vi "Timing_Main.vi"(8 "error in (no error)":errorcluster) -> (0 "error out":errorcluster)   [LabVIEW 2013]
doc: "This is Top Level VI for Timing Module. You can communicate with this module using its API. Communication is made based on queue. This module has not User Interface so I chase State Machine architecture."
uses:
  General/Controls/#TD_General_CommunicationQueueStates_Enum.ctl
  Private controls/#TD_Timing_InnerData_Cluster.ctl
  Private controls/#TD_Timing_ModuleStates_Enum.ctl
  Private controls/#TD_Timing_ModuleData_Cluster.ctl
  General/Controls/#TD_General_FromWho_Enum.ctl
  Private controls/#TD_Timing_Timers_Enum.ctl
  Private controls/#TD_Timing_TimerData_Cluster.ctl
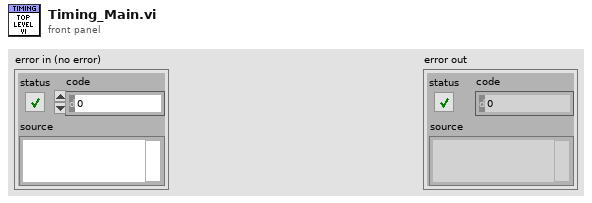
[diagram p1: front panel]
types:
  T1 = typedef "#TD_General_CommunicationQueueStates_Enum.ctl" = enum16{"ERROR_Default", "Obtain", "GetRef", "Enqueue", "EnqueueAtOpp", "GetStatus", "Release"}
  T2 = typedef "#TD_General_FromWho_Enum.ctl" = enum16{"ERROR_Default", "UserConsole", "DisplayConsole", "SensorInterface", "Controller", "Database", "Timing", "ErrorHandling"}
  T3 = typedef "#TD_Timing_ModuleStates_Enum.ctl" = enum16{"ERROR_Default", "Init", "Close", "ErrorHandling", "ResetTimer", "CheckTime", "StopTiming"}
  T4 = typedef "#TD_Timing_ModuleData_Cluster.ctl" = cluster{"Action":T3, "Data":variant}
  T5 = typedef "#TD_General_IntermoduleData_Cluster.ctl" = cluster{"Sender":T2, "ModuleData":variant}
  T6 = typedef "#TD_Timing_InnerData_Cluster.ctl" = cluster{"Sth":bool, "TimersData":T7[]}
  T7 = typedef "#TD_Timing_TimerData_Cluster.ctl" = cluster{"Timer":T8, "StartTime":timestamp, "TimeToMach":dbl, "Count?":bool}
  T8 = typedef "#TD_Timing_Timers_Enum.ctl" = enum16{"Timer_01"}
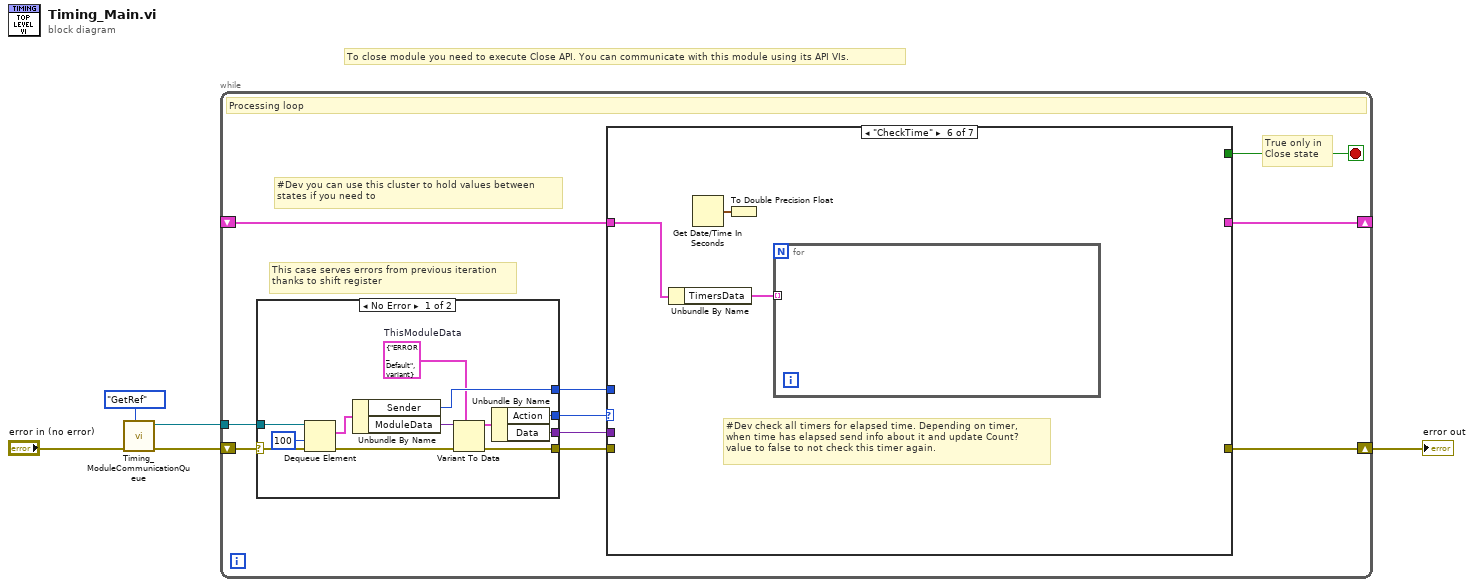
[diagram p0: block diagram]
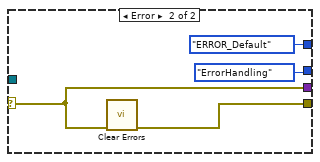
[diagram p2: hidden frame]
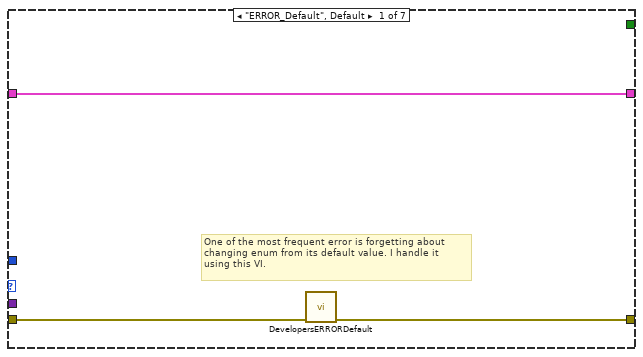
[diagram p3: hidden frame]
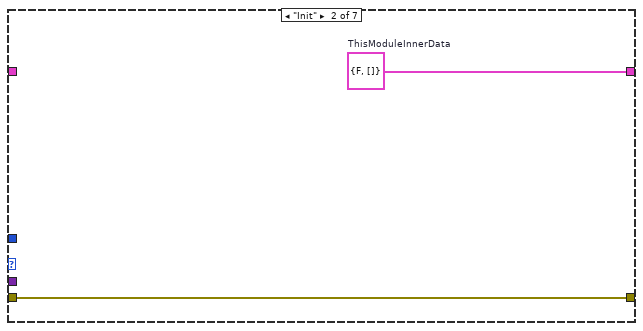
[diagram p4: hidden frame]
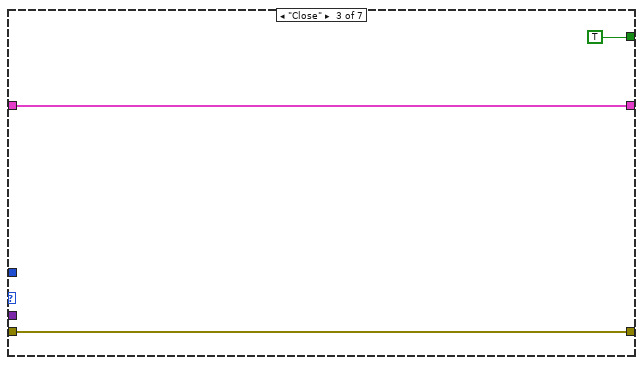
[diagram p5: hidden frame]
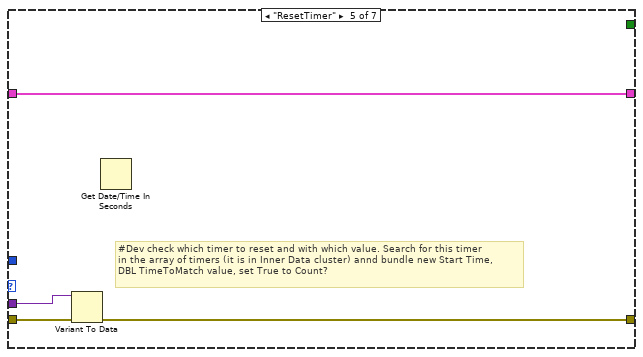
[diagram p7: hidden frame]
diagram:
  # "To close module you need to execute Close API. You can communicate with this module using its API VIs."
  n1 = call "Timing_ModuleCommunicationQueue.vi"("Action"=#TD_General_CommunicationQueueStates_Enum."GetRef", "error in (no error)"="error in (no error)") -> ("error out"=w2:errorcluster, "Ref out"=w3:refnum<queue>)  [unwired: 7 in, 1 out]
  n2 = while {
    tunnel: w3 -> [w14]
    shift-right: [w7] -> w1
    shift-left: w2 -> [w15]
    shift-right: [w13] -> _
    shift-left: _ -> [w12]
    stop <- w6 stop-if-true
    # "True only in \nClose state"
    # "#Dev you can use this cluster to hold values between \nstates if you need to"
    # "This case serves errors from previous iteration \nthanks to shift register"
    # "Processing loop"
    n3 = case shown="No Error" w15 {
      selector: w15 -> [w27 w31]
      tunnel: w14 -> [w26 _]
      tunnel: [w22 #TD_General_FromWho_Enum."ERROR_Default" ("Sender")] -> w11
      tunnel: [w19 #TD_Timing_ModuleStates_Enum."ErrorHandling" ("Action")] -> w10
      tunnel: [w18 w31] -> w9
      tunnel: [w17 w30] -> w8
      frame No Error {
        w21 = T4 {"Action"=enum."ERROR_Default", "Data"=variant}  # ThisModuleData
        n4 = Dequeue Element(queue=w26, timeout in ms (-1)=100, error in (no error)=w27) -> (element=w25:T5, error out=w23:errorcluster)  [unwired: 2 out]
        n5 = Unbundle By Name(w25) -> ("Sender"=w22:T2, "ModuleData"=w24:variant)
        n6 = Variant To Data(error in=w23, type=w21, Variant=w24) -> (data=w20:T4, error out=w17:errorcluster)
        n7 = Unbundle By Name(w20) -> ("Action"=w19:T3, "Data"=w18:variant)
      }
      frame Error {
        n8 = call <vilib>:"Clear Errors.vi"("error in (no error)"=w31) -> ("error out"=w30:errorcluster)  [unwired: 5 in, 1 out]
      }
    }
    n9 = case shown="\"CheckTime\"" w10 {
      tunnel: [w34 w36 w38 w41 w42 _ _] -> w13
      tunnel: w12 -> [w34 _ w38 w41 w42 w48 _]
      tunnel: w11 -> [_ _ _ _ _ _ _]
      tunnel: w9 -> [_ _ _ _ w44 _ _]
      tunnel: w8 -> [w33 w35 w37 w40 w45 _ _]
      tunnel: [w32 w35 w37 w40 w43 _ _] -> w7
      tunnel: [_ _ TRUE _ _ _ _] -> w6
      frame "ERROR_Default", Default {
        # "One of the most frequent error is forgetting about \nchanging enum from its default value. I handle it \nusing this VI."
        n10 = call "DevelopersERRORDefault.vi"("error in (no error)"=w33) -> ("error out"=w32:errorcluster)  [unwired: 10 in]
      }
      frame "Init" {
        w36 = T6 {"Sth"=FALSE, "TimersData"=[]}  # ThisModuleInnerData
      }
      frame "Close" {
      }
      frame "ErrorHandling" {
        # "#Dev take some actions to handle the error \nand inform central Error Handling Module \nabout this error using Error Handling Module \nAPI"
      }
      frame "ResetTimer" {
        # "#Dev check which timer to reset and with which value. Search for this timer \nin the array of timers (it is in Inner Data cluster) annd bundle new Start Time, \nDBL TimeToMatch value, set True to Count?"
        n11 = Variant To Data(error in=w45, Variant=w44) -> (error out=w43:errorcluster)  [unwired: 1 in, 1 out]
        n12 = Get Date/Time In Seconds() -> ()  [unwired: 1 out]
      }
      frame "CheckTime" {
        # "#Dev check all timers for elapsed time. Depending on timer, \nwhen time has elapsed send info about it and update Count? \nvalue to false to not check this timer again."
        n13 = Unbundle By Name(w48) -> ("TimersData"=w47:T7[])
        n14 = Get Date/Time In Seconds() -> (seconds since 1Jan1904=w46:timestamp)
        n15 = To Double Precision Float(number=w46) -> ()  [unwired: 1 out]
        n16 = for {
          tunnel: w47 -> [_] mode=indexing
        }
      }
      frame "StopTiming" {
        # "#Dev if someone ordered to stop timing then bundle \nFalse to Count? vaue in TimerData cluster for this specific \ntimer."
      }
    }
  }
  "error out" <- w1
